vi "Add Array Elements PtByPt.vi"(2 "initialize":bool, 3 "sample length":i32=100, 5 "input data point":dbl format="%0.2f") -> (0 "error":i32, 1 "sum":dbl format="%0.2f")   [LabVIEW 2020, in "NI_PtbyPt.lvlib"]
doc: "Returns the sum of all elements determined by <B>sample length</B>."
uses:
  <vilib>/ptbypt/NI_PtbyPt.lvlib
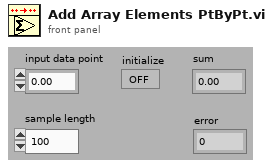
[diagram p1: front panel]
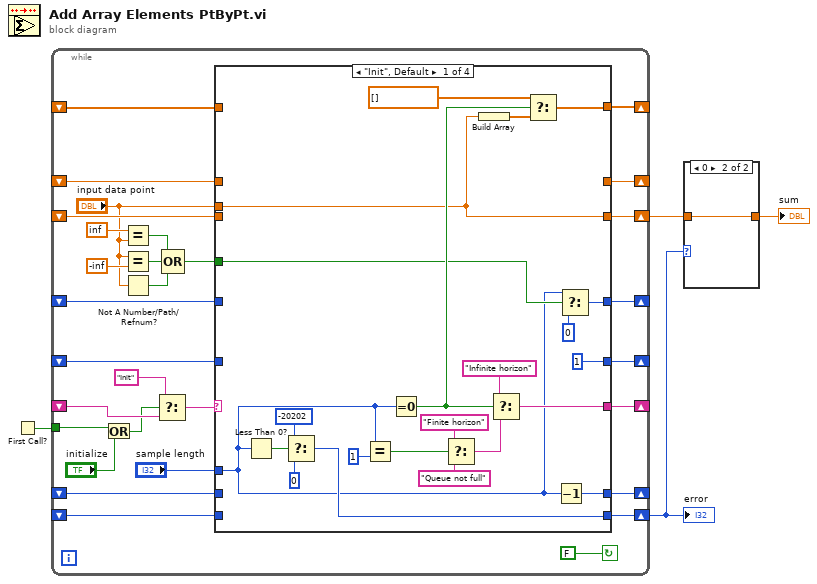
[diagram p0: block diagram]
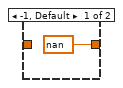
[diagram p2: hidden frame]
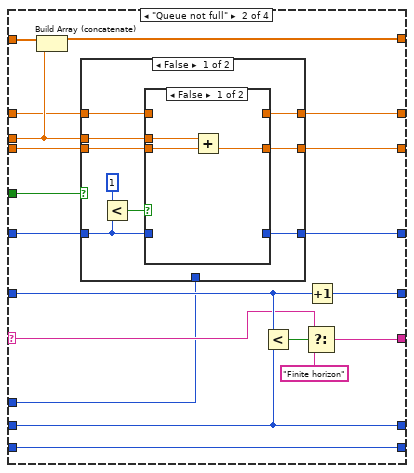
[diagram p3: hidden frame]
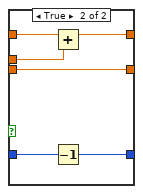
[diagram p4: hidden frame]
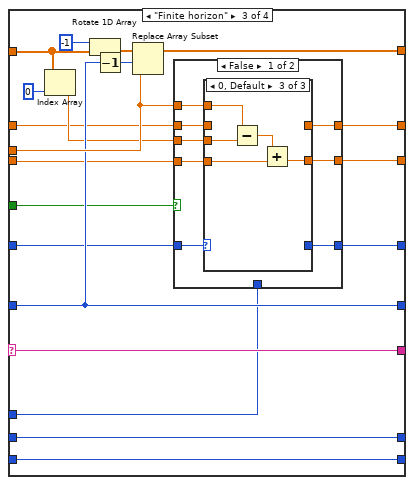
[diagram p6: hidden frame]
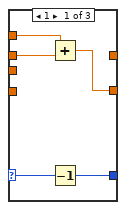
[diagram p7: hidden frame]
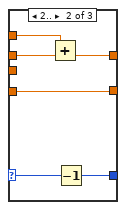
[diagram p8: hidden frame]
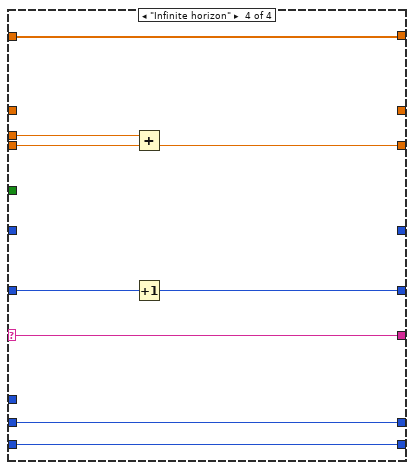
[diagram p10: hidden frame]
diagram:
  n1 = First Call?() -> (First Call?: T/F=w4:bool)
  n2 = while {
    shift-left: _ -> [w18]
    shift-right: [w19] -> _
    tunnel: w4 -> [w22]
    shift-left: _ -> [w26]
    shift-right: [w25] -> _
    shift-left: _ -> [w28]
    shift-right: [w29] -> _
    shift-left: _ -> [w30]
    shift-right: [w31] -> w2
    shift-left: _ -> [w34]
    shift-right: [w27] -> _
    shift-right: [w11] -> w3
    shift-left: _ -> [w10]
    shift-right: [w8] -> _
    shift-left: _ -> [w7]
    shift-right: [w6] -> _
    shift-left: _ -> [w5]
    stop <- FALSE continue-if-true
    n3 = Or(x=w22, y="initialize") -> (x .or. y?=w20:bool)
    n4 = Equal?(x=inf, y="input data point") -> (x = y?=w15:bool)
    n5 = Equal?(x="input data point", y=-inf) -> (x = y?=w16:bool)
    n6 = Not A Number/Path/Refnum?(number/path/refnum="input data point") -> (NaN/Path/Refnum?=w14:bool)
    n7 = Select(t="Init", s=w20, f=w34) -> (s? t:f=w32:string)
    n8 = Compound Arithmetic op=OR(w15, w16, w14) -> (w9:bool)
    n9 = case shown="\"Init\", Default" w32 {
      selector: w32 -> [_ w68 w106 w146]
      tunnel: [w47 w71 w105 w148] -> w31
      tunnel: w30 -> [_ w72 w104 w150]
      tunnel: "input data point" -> [w47 w73 w112 w149]
      tunnel: [1 w64 w110 w143] -> w29
      tunnel: w28 -> [_ w70 w110 w147]
      tunnel: [w49 w66 w106 w146] -> w27
      tunnel: w26 -> [_ w75 w107 w145]
      tunnel: [w44 w74 w109 w145] -> w25
      tunnel: "sample length" -> [w37 w58 w97 _]
      tunnel: [w40 w65 w103 w144] -> w19
      tunnel: w18 -> [_ w65 w103 w144]
      tunnel: [w39 w57 w96 w142] -> w11
      tunnel: w10 -> [_ w57 w96 w142]
      tunnel: w9 -> [w38 w63 w102 _]
      tunnel: [w35 w61 w99 _] -> w8
      tunnel: w7 -> [_ w62 w101 _]
      tunnel: [_ w60 w98 _] -> w6
      tunnel: w5 -> [_ w59 w100 _]
      frame "Init", Default {
        n10 = Less Than 0?(x=w37) -> (x < 0?=w43:bool)
        n11 = Select(t=-20202, s=w43, f=0) -> (s? t:f=w39:i32)
        n12 = Equal?(x=w37, y=1) -> (x = y?=w53:bool)
        n13 = Equal To 0?(x=w37) -> (x = 0?=w48:bool)
        n14 = Select(t="Finite horizon", s=w53, f="Queue not full") -> (s? t:f=w51:string)
        n15 = Build Array(w47) -> (w46:dbl[])
        n16 = Select(t="Infinite horizon", s=w48, f=w51) -> (s? t:f=w49:string)
        n17 = Select(t=dbl[] [], s=w48, f=w46) -> (s? t:f=w44:dbl[])
        n18 = Decrement(x=w37) -> (x-1=w40:i32)
        n19 = Select(t=w37, s=w38, f=0) -> (s? t:f=w35:i32)
      }
      frame "Queue not full" {
        n20 = Build Array (concatenate)(w75, w73) -> (w74:dbl[])
        n21 = case shown="False" w63 {
          tunnel: w73 -> [w84 w95]
          tunnel: w72 -> [w83 _]
          tunnel: [w82 w95] -> w71
          tunnel: w62 -> [w79 _]
          tunnel: [w78 w94] -> w61
          tunnel: [w77 _] -> w60
          tunnel: w59 -> [w76 _]
          tunnel: w58 -> [_ w94]
          frame False {
            n22 = Less?(x=1, y=w79) -> (x < y?=w80:bool)
            n23 = case shown="False" w80 {
              tunnel: w84 -> [w87 w89]
              tunnel: w83 -> [w86 w88]
              tunnel: [w85 w88] -> w82
              tunnel: w79 -> [_ w93]
              tunnel: [_ w92] -> w78
              tunnel: [_ w91] -> w77
              tunnel: w76 -> [_ w90]
              frame False {
                n24 = Add(x=w87, y=w86) -> (x+y=w85:dbl)
              }
              frame True {
                n25 = Add(x=w90, y=w89) -> (x+y=w91:dbl)
                n26 = Decrement(x=w93) -> (x-1=w92:i32)
              }
            }
          }
          frame True {
          }
        }
        n27 = Less?(x=w70, y=w65) -> (x < y?=w69:bool)
        n28 = Select(t=w68, s=w69, f="Finite horizon") -> (s? t:f=w66:string)
        n29 = Increment(x=w70) -> (x+1=w64:i32)
      }
      frame "Finite horizon" {
        n30 = Index Array(array=w107, index=0 ("Index")) -> (element=w108:dbl)
        n31 = Rotate 1D Array(1:w107, 2:i16 -1 ("n")) -> (0:w113:dbl[])
        n32 = Decrement(x=w110) -> (x-1=w111:i32)
        n33 = Replace Array Subset(array=w113, new element=w112, index=w111) -> (w109:dbl[])
        n34 = case shown="False" w102 {
          tunnel: w112 -> [w123 w140]
          tunnel: w108 -> [w122 _]
          tunnel: [w121 w140] -> w105
          tunnel: w104 -> [w120 _]
          tunnel: w101 -> [w119 _]
          tunnel: w100 -> [w118 _]
          tunnel: [w117 w141] -> w99
          tunnel: [w116 _] -> w98
          tunnel: w97 -> [_ w141]
          frame False {
            n35 = case shown="0, Default" w119 {
              selector: w119 -> [w127 w130 _]
              tunnel: w123 -> [w124 w134 w139]
              tunnel: w122 -> [_ _ w138]
              tunnel: [w128 w129 w137] -> w121
              tunnel: w120 -> [_ w129 w135]
              tunnel: w118 -> [w125 w132 _]
              tunnel: [w126 w131 _] -> w117
              tunnel: [_ w133 _] -> w116
              frame 1 {
                n36 = Add(x=w124, y=w125) -> (x+y=w128:dbl)
                n37 = Decrement(x=w127) -> (x-1=w126:i32)
              }
              frame 2.. {
                n38 = Add(x=w134, y=w132) -> (x+y=w133:dbl)
                n39 = Decrement(x=w130) -> (x-1=w131:i32)
              }
              frame 0, Default {
                n40 = Subtract(x=w139, y=w138) -> (x-y=w136:dbl)
                n41 = Add(x=w136, y=w135) -> (x+y=w137:dbl)
              }
            }
          }
          frame True {
          }
        }
      }
      frame "Infinite horizon" {
        n42 = Add(x=w149, y=w150) -> (x+y=w148:dbl)
        n43 = Increment(x=w147) -> (x+1=w143:i32)
      }
    }
  }
  "error" <- w3
  n44 = case shown="0" w3 {
    tunnel: w2 -> [_ w152]
    tunnel: [nan ("input data point") w152] -> w1
    frame -1, Default {
    }
    frame 0 {
    }
  }
  "sum" <- w1
